vi "Open Image Sequence.vi"(8 "error in (no error)":errorcluster, 11 "Frame Grabber Data In":T1={"Camera Session"="", "Frame"=refnum, "AVI Refnum"=refnum, "Codecs"=[], "Frame number"=0, "Tracking File Refnum"=refnum, "Tick Count"=0, "Probe Object"=refnum, "Playback Probe Data"=[], "Rigid Body"={"Position"={"x (mm)"=0.0, "y (mm)"=0.0, "z (mm)"=0.0}, "Orientation"={"Pitch (rad)"=0.0, "Yaw (rad)"=0.0, "Roll (rad)"=0.0}, "Quaternion"={"qx"=0.0, "qy"=0.0, "qz"=0.0, "qw"=0.0}, "Tracked?"=FALSE}, "Total no frames playback"=0, "Video FPS"=0.0, "Camera connected?"=FALSE, "Scene"=refnum, "Cropped Frame"=refnum, "Tracker FPS"=0.0, "Crop ROI"=[], "Presentation Values"=[], "Elapsed time (ms)"=0, "Camera frames playback"=0, "Refnums"={"Live Refnum"=refnum, "Record Refnum"=refnum, "Playback Refnum"=refnum, "Frame Slider Refnum"=refnum, "Pause Refnum"=refnum, "Home Refnum"=refnum, "Set Crop Refnum"=refnum, "Clear Crop Refnum"=refnum, "stop refnum"=refnum, "Playback Rate Refnum"=refnum, "Presentation Refnum"=refnum, "Crop Time Frame Slider Refnum"=refnum, "Cancel Save Refnum"=refnum, "Reverse Playback Refnum"=refnum, "Recording Settings Refnum"=refnum, "Continuous Playback Refnum"=refnum, "Annotation Refnum"=refnum, "Export All Refnum"=refnum, "Export List Refnum"=refnum, "Fill List Refnum"=refnum, "Save Crop Refnum"=refnum, "Skip Forward Refnum"=refnum, "Skip Backward Refnum"=refnum, "Single Annotation Refnum"=refnum, "Load Video Refnum"=refnum, "Set Start Refnum"=refnum, "Set End Refnum"=refnum, "Add to List Refnum"=refnum, "List of Annotations Refnum"=refnum, "Camera Frame Refnum"=refnum, "Load Image Refnum"=refnum, "Saving Refnum"=refnum}, "Dimensions"={"Probe Dimensions"={"Probe Width"=0.0, "Probe Depth"=1.0, "Probe Height"=0.0}, "Room Dimensions"={"Room Width"=0.0, "Room Depth"=0.0, "Room Height"=0.0}}, "Playback Data As Strings"=[], "Cropped Tracking File Refnum"=refnum, "Cropped AVI Refnum"=refnum, "Header"=[], "Total euclidian distance"=0.0, "Annotation File Path"=path "", "Playback File Path"=path "", "Size per frame"=0.0, "Ground Truth File Refnum"=refnum, "Annotation Array"=[], "Annotation TIFFs Folder"=path "", "overwriting open file?"=FALSE, "Image Sequence"=[], "Video/Image Flag"=enum."Playback Video Frame", "Image sequence?"=FALSE, "Image sequence filenames"=[], "Mask"=refnum}) -> (0 "error out":errorcluster, 1 "opened?":bool, 2 "directory":path, 3 "Frame Grabber Data Out":T1={"Camera Session"="", "Frame"=refnum, "AVI Refnum"=refnum, "Codecs"=[], "Frame number"=0, "Tracking File Refnum"=refnum, "Tick Count"=0, "Probe Object"=refnum, "Playback Probe Data"=[], "Rigid Body"={"Position"={"x (mm)"=0.0, "y (mm)"=0.0, "z (mm)"=0.0}, "Orientation"={"Pitch (rad)"=0.0, "Yaw (rad)"=0.0, "Roll (rad)"=0.0}, "Quaternion"={"qx"=0.0, "qy"=0.0, "qz"=0.0, "qw"=0.0}, "Tracked?"=FALSE}, "Total no frames playback"=0, "Video FPS"=0.0, "Camera connected?"=FALSE, "Scene"=refnum, "Cropped Frame"=refnum, "Tracker FPS"=0.0, "Crop ROI"=[], "Presentation Values"=[], "Elapsed time (ms)"=0, "Camera frames playback"=0, "Refnums"={"Live Refnum"=refnum, "Record Refnum"=refnum, "Playback Refnum"=refnum, "Frame Slider Refnum"=refnum, "Pause Refnum"=refnum, "Home Refnum"=refnum, "Set Crop Refnum"=refnum, "Clear Crop Refnum"=refnum, "stop refnum"=refnum, "Playback Rate Refnum"=refnum, "Presentation Refnum"=refnum, "Crop Time Frame Slider Refnum"=refnum, "Cancel Save Refnum"=refnum, "Reverse Playback Refnum"=refnum, "Recording Settings Refnum"=refnum, "Continuous Playback Refnum"=refnum, "Annotation Refnum"=refnum, "Export All Refnum"=refnum, "Export List Refnum"=refnum, "Fill List Refnum"=refnum, "Save Crop Refnum"=refnum, "Skip Forward Refnum"=refnum, "Skip Backward Refnum"=refnum, "Single Annotation Refnum"=refnum, "Load Video Refnum"=refnum, "Set Start Refnum"=refnum, "Set End Refnum"=refnum, "Add to List Refnum"=refnum, "List of Annotations Refnum"=refnum, "Camera Frame Refnum"=refnum, "Load Image Refnum"=refnum, "Saving Refnum"=refnum}, "Dimensions"={"Probe Dimensions"={"Probe Width"=0.0, "Probe Depth"=1.0, "Probe Height"=0.0}, "Room Dimensions"={"Room Width"=0.0, "Room Depth"=0.0, "Room Height"=0.0}}, "Playback Data As Strings"=[], "Cropped Tracking File Refnum"=refnum, "Cropped AVI Refnum"=refnum, "Header"=[], "Total euclidian distance"=0.0, "Annotation File Path"=path "", "Playback File Path"=path "", "Size per frame"=0.0, "Ground Truth File Refnum"=refnum, "Annotation Array"=[], "Annotation TIFFs Folder"=path "", "overwriting open file?"=FALSE, "Image Sequence"=[], "Video/Image Flag"=enum."Playback Video Frame", "Image sequence?"=FALSE, "Image sequence filenames"=[], "Mask"=refnum}, 4 "frame(s)":i32, 5 "sequence":bool)   [LabVIEW 2017]
uses:
  Controls/Frame Grabber Data.ctl
  <vilib>/userdefined/High Color/IMAQdx.ctl
  <vilib>/vision/Image Controls.llb/IMAQ Image.ctl
  <vilib>/vision/Avi.llb/IMAQ AVI2 Refnum.ctl
  Controls/Rigid Body Info.ctl
  Controls/Position.ctl
  Controls/Orientation.ctl
  Controls/Refnums.ctl
  Controls/Recording Settings.ctl
  Controls/Operator Settings.ctl
  Controls/Operator.ctl
  Controls/Patient Settings.ctl
  Controls/Dimensions.ctl
  Controls/Room Dimensions.ctl
  Controls/Crop Video State.ctl
panel:
  out "filename(s)":string[](array[string])
  out "Image Sequence":T3[](array[plugin-control])
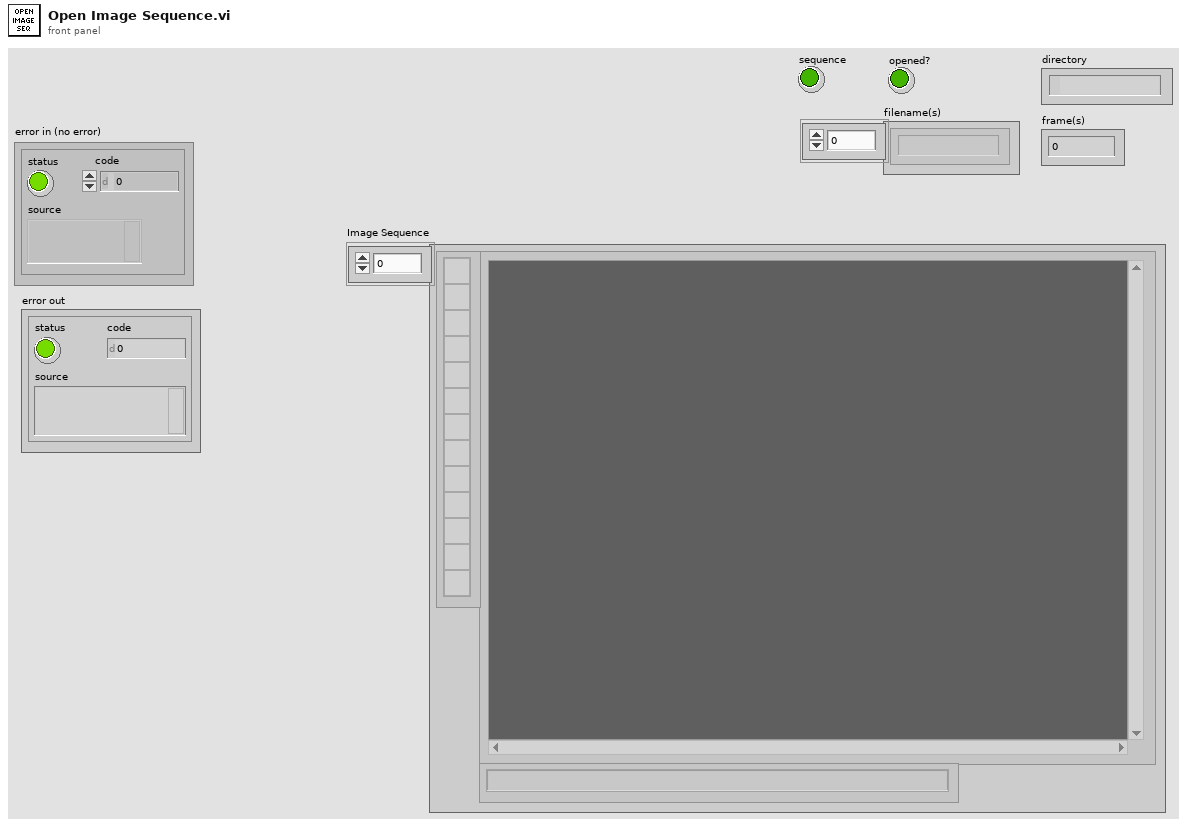
[diagram p1: front panel]
types:
  T1 = typedef "Frame Grabber Data.ctl" = cluster{"Camera Session":T2, "Frame":T3, "AVI Refnum":T4, "Codecs":string[], "Frame number":u32, "Tracking File Refnum":refnum<file>, "Tick Count":u32, "Probe Object":refnum<vi>, "Playback Probe Data":dbl[][], "Rigid Body":T5, "Total no frames playback":i32, "Video FPS":dbl, "Camera connected?":bool, "Scene":refnum<vi>, "Cropped Frame":T3, "Tracker FPS":dbl, "Crop ROI":i32[], "Presentation Values":string[], "Elapsed time (ms)":u32, "Camera frames playback":u32, "Refnums":T8, "Dimensions":T9, "Playback Data As Strings":string[][], "Cropped Tracking File Refnum":refnum<file>, "Cropped AVI Refnum":T4, "Header":string[], "Total euclidian distance":dbl, "Annotation File Path":path, "Playback File Path":path, "Size per frame":dbl, "Ground Truth File Refnum":refnum<file>, "Annotation Array":string[], "Annotation TIFFs Folder":path, "overwriting open file?":bool, "Image Sequence":T3[], "Video/Image Flag":T11, "Image sequence?":bool, "Image sequence filenames":string[], "Mask":T3}
  T2 = typedef "IMAQdx.ctl" = refnum<k21>
  T3 = typedef "IMAQ Image.ctl" = refnum<image>
  T4 = typedef "IMAQ AVI2 Refnum.ctl" = refnum<k20>
  T5 = typedef "Rigid Body Info.ctl" = cluster{"Position":T6, "Orientation":T7, "Quaternion":cluster{"qx":sgl, "qy":sgl, "qz":sgl, "qw":sgl}, "Tracked?":bool}
  T6 = typedef "Position.ctl" = cluster{"x (mm)":sgl, "y (mm)":sgl, "z (mm)":sgl}
  T7 = typedef "Orientation.ctl" = cluster{"Pitch (rad)":sgl, "Yaw (rad)":sgl, "Roll (rad)":sgl}
  T8 = typedef "Refnums.ctl" = cluster{"Live Refnum":refnum<vi>, "Record Refnum":refnum<vi>, "Playback Refnum":refnum<vi>, "Frame Slider Refnum":refnum<vi>, "Pause Refnum":refnum<vi>, "Home Refnum":refnum<vi>, "Set Crop Refnum":refnum<vi>, "Clear Crop Refnum":refnum<vi>, "stop refnum":refnum<vi>, "Playback Rate Refnum":refnum<vi>, "Presentation Refnum":refnum<vi>, "Crop Time Frame Slider Refnum":refnum<vi>, "Cancel Save Refnum":refnum<vi>, "Reverse Playback Refnum":refnum<vi>, "Recording Settings Refnum":refnum<vi>, "Continuous Playback Refnum":refnum<vi>, "Annotation Refnum":refnum<vi>, "Export All Refnum":refnum<vi>, "Export List Refnum":refnum<vi>, "Fill List Refnum":refnum<vi>, "Save Crop Refnum":refnum<vi>, "Skip Forward Refnum":refnum<vi>, "Skip Backward Refnum":refnum<vi>, "Single Annotation Refnum":refnum<vi>, "Load Video Refnum":refnum<vi>, "Set Start Refnum":refnum<vi>, "Set End Refnum":refnum<vi>, "Add to List Refnum":refnum<vi>, "List of Annotations Refnum":refnum<vi>, "Camera Frame Refnum":refnum<vi>, "Load Image Refnum":refnum<vi>, "Saving Refnum":refnum<vi>}
  T9 = typedef "Dimensions.ctl" = cluster{"Probe Dimensions":cluster{"Probe Width":sgl, "Probe Depth":sgl, "Probe Height":sgl}, "Room Dimensions":T10}
  T10 = typedef "Room Dimensions.ctl" = cluster{"Room Width":dbl, "Room Depth":dbl, "Room Height":dbl}
  T11 = typedef "Crop Video State.ctl" = enum16{"Init", "Wait", "Load Image", "Load Video", "Play/Pause", "Playback Video Frame", "Display Image", "Save Image Sequence", "Save Video", "Export List", "Export All", "Close", "Set Crop Area", "Reset Crop Area", "Crop Inside", "Crop Outside", "Multi-Crop", "Re-Open Files", "Annotate Frame", "Annotate Clip", "Add to List", "Fill List", "Set Start", "Set End", "Error Handling", "Shutdown"}
  T12 = typedef "Image Type" = u32
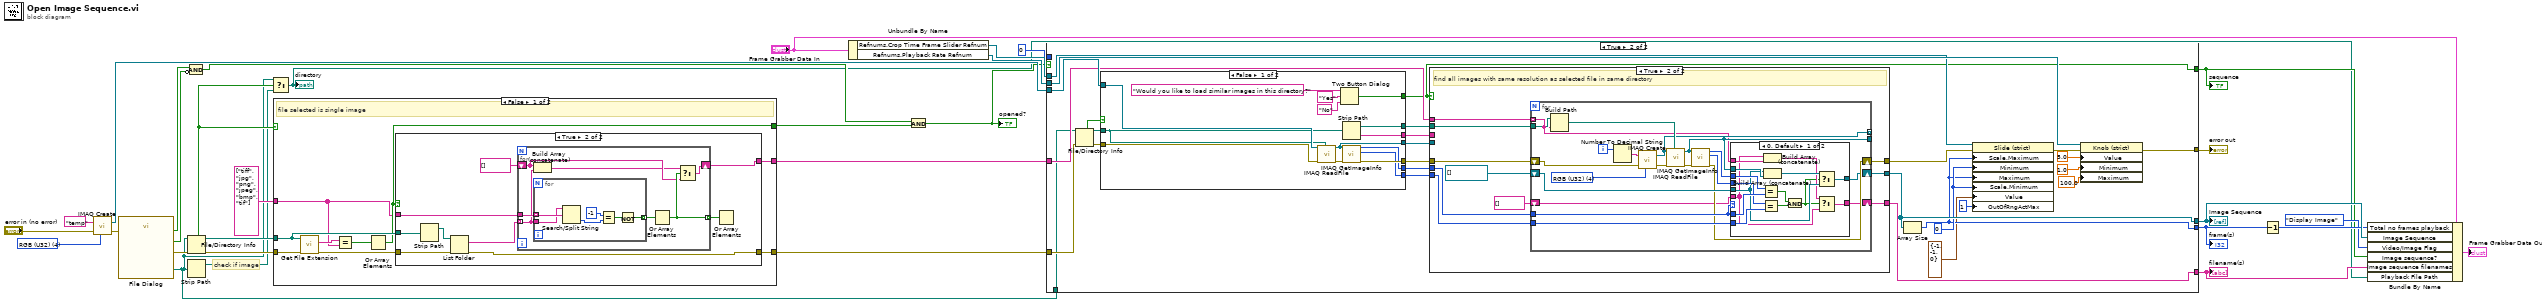
[diagram p0: block diagram]
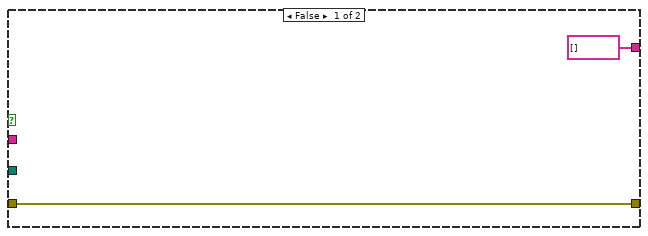
[diagram p2: hidden frame]
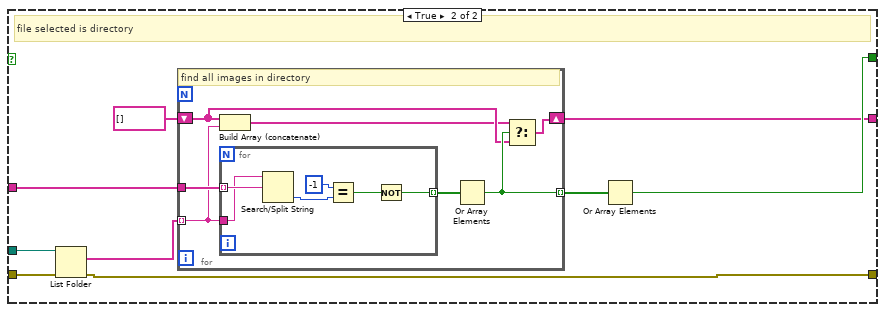
[diagram p3: hidden frame]
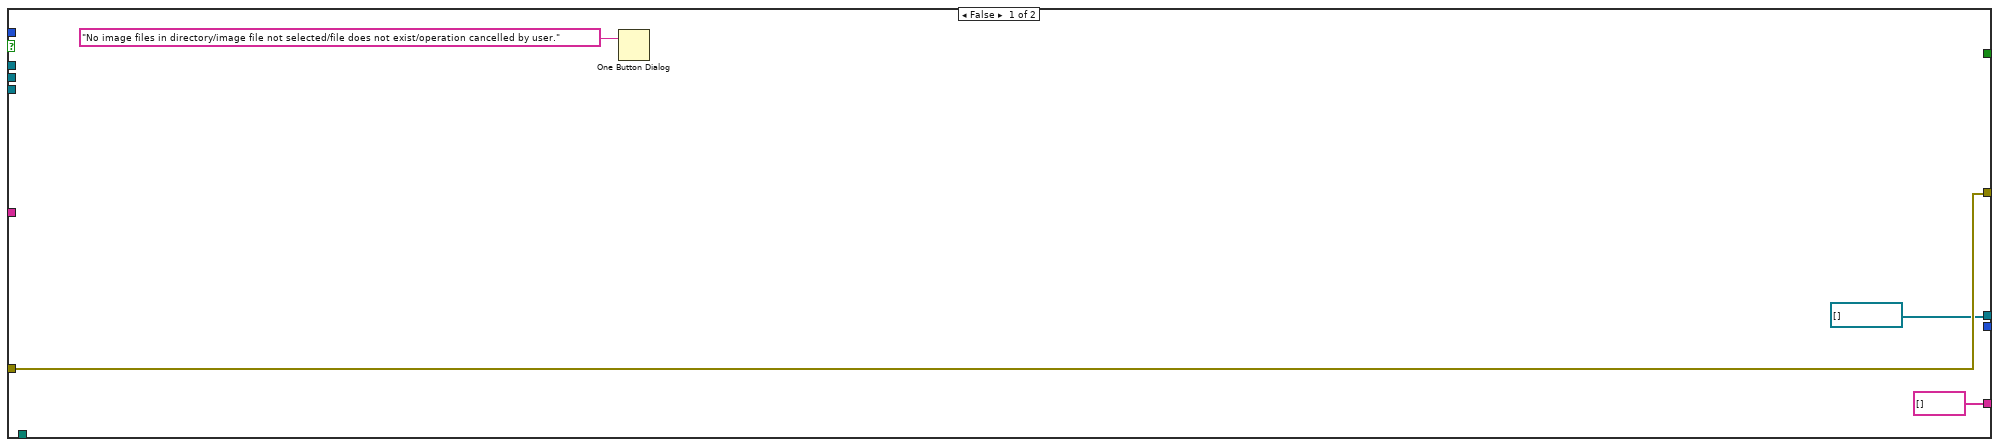
[diagram p4: hidden frame]
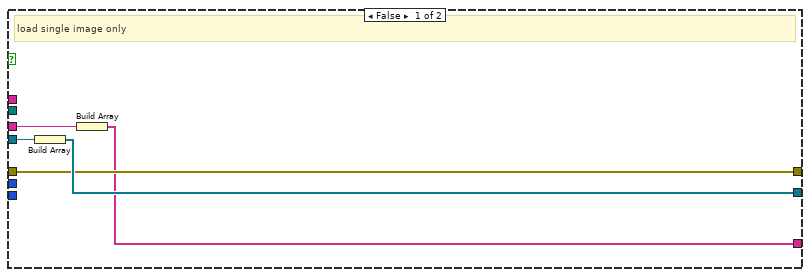
[diagram p5: hidden frame]
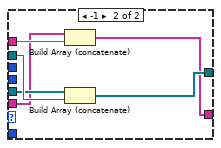
[diagram p6: hidden frame]
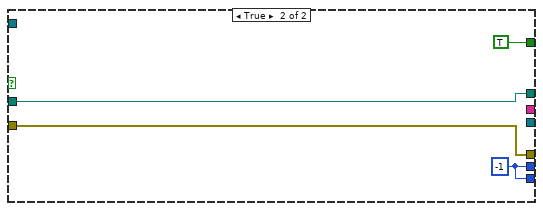
[diagram p7: hidden frame]
diagram:
  w31 = T12 4 items=["Grayscale (U8)", "Grayscale (I16)", "Grayscale (SGL)", "Complex (CSG)", "RGB (U32)", "HSL (U32)", "RGB (U64)", "Grayscale (U16)"] ("Image Type")
  # "check if image"
  n1 = call "IMAQ Create"("Image Name"="temp", "Image Type"=w31, "error in (no error)"="error in (no error)") -> ("New Image"=w29:T3, "error out"=w32:errorcluster)  [unwired: 2 in]
  n2 = call "File Dialog"("error in"=w32) -> ("selected path"=w1:path, "exists"=w26:bool, "cancelled"=w28:bool, "error out"=w17:errorcluster)  [unwired: 11 in]
  n3 = File/Directory Info(path=w1, error in=w17) -> (path out=w16:path, directory=w6:bool, error out=w14:errorcluster)  [unwired: 4 out]
  n4 = Strip Path(path=w1) -> (stripped path=w5:path)  [unwired: 1 out]
  n5 = Compound Arithmetic op=AND(w26, invert w28) -> (w27:bool)
  n6 = Select(t=w1, s=w6, f=w5) -> (s? t:f=w2:path)
  "directory" <- w2
  n7 = case shown="False" w6 {
    tunnel: w16 -> [w38 w74]
    tunnel: string[] ["tiff", "jpg", "png", "jpeg", "bmp", "tif"] -> [w35 w69]
    tunnel: w14 -> [w39 w73]
    tunnel: [w34 w68] -> w12
    tunnel: [w36 w70] -> w13
    tunnel: [w33 w66] -> w11
    frame False {
      # "file selected is single image"
      n8 = call <vilib>:"Get File Extension.vi"("error in (no error)"=w39, "file"=w38) -> ("error out"=w37:errorcluster, "lowercase file extension"=w40:string)  [unwired: 5 in, 3 out]
      n9 = Equal?(x=w40, y=w35) -> (x = y?=w41:bool[])
      n10 = Or Array Elements(Boolean array=w41) -> (logical OR=w36:bool)
      n11 = case shown="True" w36 {
        tunnel: w38 -> [_ w52]
        tunnel: w37 -> [w43 w46]
        tunnel: w35 -> [_ w48]
        tunnel: [w43 w45] -> w34
        tunnel: [string[] [] w44] -> w33
        frame False {
        }
        frame True {
          n12 = Strip Path(path=w52) -> (stripped path=w47:path)  [unwired: 1 out]
          n13 = List Folder(path=w47, error in=w46) -> (filenames=w50:string[], error out=w45:errorcluster)  [unwired: 2 in, 2 out]
          n14 = for {
            tunnel: w50 -> [w54] mode=indexing
            tunnel: [w59] -> w51 mode=indexing
            tunnel: w48 -> [w55]
            shift-right: [w58] -> w44
            shift-left: string[] [] -> [w57]
            n15 = Build Array (concatenate)(w57, w54) -> (w56:string[])
            n16 = for {
              tunnel: [w62] -> w53 mode=indexing
              tunnel: w55 -> [w61] mode=indexing
              tunnel: w54 -> [w60]
              n17 = Search/Split String(string=w60, search string/char (-)=w61) -> (offset of match=w65:i32)  [unwired: 1 in, 2 out]
              n18 = Equal?(x=-1, y=w65) -> (x = y?=w63:bool)
              n19 = Not(x=w63) -> (.not. x?=w62:bool)
            }
            n20 = Or Array Elements(Boolean array=w53) -> (logical OR=w59:bool)
            n21 = Select(t=w56, s=w59, f=w57) -> (s? t:f=w58:string[])
          }
          n22 = Or Array Elements(Boolean array=w51) -> ()  [unwired: 1 out]
        }
      }
    }
    frame True {
      # "file selected is directory"
      n23 = List Folder(path=w74, error in=w73) -> (filenames=w72:string[], error out=w68:errorcluster)  [unwired: 2 in, 2 out]
      n24 = for {
        tunnel: w72 -> [w76] mode=indexing
        tunnel: [w81] -> w71 mode=indexing
        tunnel: w69 -> [w77]
        shift-right: [w80] -> w66
        shift-left: string[] [] -> [w79]
        # "find all images in directory"
        n25 = Build Array (concatenate)(w79, w76) -> (w78:string[])
        n26 = for {
          tunnel: [w84] -> w75 mode=indexing
          tunnel: w77 -> [w83] mode=indexing
          tunnel: w76 -> [w82]
          n27 = Search/Split String(string=w82, search string/char (-)=w83) -> (offset of match=w87:i32)  [unwired: 1 in, 2 out]
          n28 = Equal?(x=-1, y=w87) -> (x = y?=w85:bool)
          n29 = Not(x=w85) -> (.not. x?=w84:bool)
        }
        n30 = Or Array Elements(Boolean array=w75) -> (logical OR=w81:bool)
        n31 = Select(t=w78, s=w81, f=w79) -> (s? t:f=w80:string[])
      }
      n32 = Or Array Elements(Boolean array=w71) -> (logical OR=w70:bool)
    }
  }
  n33 = Unbundle By Name("Frame Grabber Data In") -> ("Refnums.Crop Time Frame Slider Refnum"=w19:refnum<vi>, "Refnums.Playback Rate Refnum"=w20:refnum<vi>)
  n34 = And(x=w27, y=w13) -> (x .and. y?=w3:bool)
  "opened?" <- w3
  n35 = case shown="True" w3 {
    tunnel: w12 -> [w91 w119]
    tunnel: w29 -> [_ w113]
    tunnel: [w91 w103] -> w24
    tunnel: [T3[] [] w108] -> w22
    tunnel: [string[] [] w110] -> w7
    tunnel: [_ w93] -> w4
    tunnel: w20 -> [_ w106]
    tunnel: w19 -> [_ w102]
    tunnel: u32 0 ("Value") -> [_ _]
    tunnel: [_ w99] -> w10
    tunnel: w11 -> [_ w96]
    tunnel: w1 -> [_ w92]
    frame False {
      n36 = One Button Dialog(message="No image files in directory/image file not selected/file does not exist/operation cancelled by user.") -> ()  [unwired: 1 in, 1 out]
    }
    frame True {
      w100 = 0 ("Data Entry Limits:Minimum")
      n37 = File/Directory Info(path=w92, error in=w119) -> (path out=w116:path, directory=w97:bool, error out=w118:errorcluster)  [unwired: 4 out]
      n38 = case shown="False" w97 {
        tunnel: w118 -> [w176 w193]
        tunnel: [w187 w193] -> w117
        tunnel: [w178 TRUE ("T button?")] -> w93
        tunnel: w116 -> [w177 w191]
        tunnel: [w180 w191] -> w111
        tunnel: [w186 w192] -> w115
        tunnel: [w185 w192] -> w114
        tunnel: w113 -> [w184 _]
        tunnel: [w183 _] -> w112
        tunnel: [w179 _] -> w109
        frame False {
          n39 = call "IMAQ ReadFile"("File Path"=w177, "error in (no error)"=w176, "Image"=w184) -> ("error out"=w188:errorcluster, "Image Out"=w183:T3)  [unwired: 4 in, 3 out]
          n40 = Two Button Dialog(message="Would you like to load similar images in this directory?", 1:"No" ("F button name (\"Cancel\")"), 2:"Yes" ("T button name (\"OK\")")) -> (T button?=w178:bool)
          n41 = Strip Path(path=w177) -> (stripped path=w180:path, name=w179:string)
          n42 = call "IMAQ GetImageInfo"("error in (no error)"=w188, "Image"=w183) -> ("error out"=w187:errorcluster, "Y Resolution"=w186:i32, "X Resolution"=w185:i32)  [unwired: 2 in, 5 out]
        }
        frame True {
          w192 = -1 ("X Resolution")
        }
      }
      n43 = case shown="True" w93 {
        tunnel: w117 -> [w122 w125]
        tunnel: w111 -> [_ w126]
        tunnel: w115 -> [_ w134]
        tunnel: w114 -> [_ w133]
        tunnel: [w122 w131] -> w101
        tunnel: w112 -> [w124 _]
        tunnel: [w123 w130] -> w108
        tunnel: [w120 w128] -> w110
        tunnel: w109 -> [w121 _]
        tunnel: w96 -> [_ w127]
        frame False {
          # "load single image only"
          n44 = Build Array(w124) -> (w123:T3[])
          n45 = Build Array(w121) -> (w120:string[])
        }
        frame True {
          # "find all images with same resolution as selected file in same directory"
          n46 = for {
            tunnel: w127 -> [w137] mode=indexing
            tunnel: w126 -> [w154]
            shift-right: [w139] -> w131
            shift-left: w125 -> [w144]
            tunnel: w134 -> [w147]
            tunnel: w133 -> [w149]
            tunnel: [w140] -> _ mode=indexing
            shift-right: [w138] -> w130
            shift-left: T3[] [] -> [w151]
            tunnel: [w146] -> _
            shift-right: [w136] -> w128
            shift-left: string[] [] -> [w135]
            i -> [w145]
            w142 = T12 4 items=["Grayscale (U8)", "Grayscale (I16)", "Grayscale (SGL)", "Complex (CSG)", "RGB (U32)", "HSL (U32)", "RGB (U64)", "Grayscale (U16)"] ("Image Type")
            # "find all images with same resolution as selected file"
            n47 = Build Path(base path=w154, name or relative path=w137) -> (appended path=w153:path)
            n48 = Number To Decimal String(number=w145) -> (decimal integer string=w141:string)  [unwired: 1 in]
            n49 = call "IMAQ Create"("Image Name"=w141, "Image Type"=w142, "error in (no error)"=w144) -> ("New Image"=w140:T3, "error out"=w143:errorcluster)  [unwired: 2 in]
            n50 = call "IMAQ ReadFile"("File Path"=w153, "error in (no error)"=w143, "Image"=w140) -> ("error out"=w152:errorcluster, "Image Out"=w146:T3)  [unwired: 4 in, 3 out]
            n51 = call "IMAQ GetImageInfo"("error in (no error)"=w152, "Image"=w146) -> ("error out"=w139:errorcluster, "Y Resolution"=w148:i32, "X Resolution"=w150:i32)  [unwired: 2 in, 5 out]
            n52 = case shown="0, Default" w149 {
              tunnel: w146 -> [w163 w175]
              tunnel: [w160 w174] -> w138
              tunnel: w151 -> [w161 w173]
              tunnel: w150 -> [w169 _]
              tunnel: w149 -> [w168 _]
              tunnel: w148 -> [w167 _]
              tunnel: w147 -> [w166 _]
              tunnel: w137 -> [w156 w172]
              tunnel: [w158 w171] -> w136
              tunnel: w135 -> [w155 w170]
              frame 0, Default {
                n53 = Equal?(x=w169, y=w168) -> (x = y?=w165:bool)
                n54 = Equal?(x=w167, y=w166) -> (x = y?=w164:bool)
                n55 = Build Array (concatenate)(w155, w156) -> (w159:string[])
                n56 = Build Array (concatenate)(w161, w163) -> (w162:T3[])
                n57 = And(x=w165, y=w164) -> (x .and. y?=w157:bool)
                n58 = Select(t=w162, s=w157, f=w161) -> (s? t:f=w160:T3[])
                n59 = Select(t=w159, s=w157, f=w155) -> (s? t:f=w158:string[])
              }
              frame -1 {
                n60 = Build Array (concatenate)(w170, w172) -> (w171:string[])
                n61 = Build Array (concatenate)(w173, w175) -> (w174:T3[])
              }
            }
          }
        }
      }
      n62 = Array Size(array=w108) -> (size(s)=w99:i32)
      n63 = property class="Slide (strict)"(reference=w102, error in=w101, "Scale.Maximum"=w99, "Minimum"=w100, "Maximum"=w99, "Scale.Minimum"=w100, "Value"=cluster{i32, i32, i32} {-1, -1, 0}, "OutOfRngActMax"=u8 1 ("Response to Value Outside Limits:Maximum")) -> (error out=w107:errorcluster)  [unwired: 1 out]
      n64 = property class="Knob (strict)"(reference=w106, error in=w107, "Value"=5.0, "Minimum"=1.0 ("Data Entry Limits:Maximum"), "Maximum"=100.0 ("Data Entry Limits:Minimum")) -> (error out=w103:errorcluster)  [unwired: 1 out]
    }
  }
  "Image Sequence" <- w22
  "error out" <- w24
  "sequence" <- w4
  "filename(s)" <- w7
  "frame(s)" <- w10
  n65 = Decrement(x=w10) -> (x-1=w9:i32)
  n66 = Bundle By Name(cluster="Frame Grabber Data In", "Total no frames playback"=w9, "Image Sequence"=w22, "Video/Image Flag"=Crop_Video_State."Display Image", "Image sequence?"=w4, "Image sequence filenames"=w7, "Playback File Path"=w2) -> (→"Frame Grabber Data Out":T1)
